vi "Send.vi"(8 "error in (no error)":errorcluster, 11 "BaseDriver in":refnum<class "BaseDriver.lvclass">) -> (0 "error out":errorcluster, 3 "BaseDriver out":refnum<class "BaseDriver.lvclass">)   [LabVIEW 2013, in "BaseDriver.lvclass"]
doc: "Send a message to the remote destination"
uses:
  BaseDriver.lvclass
  BaseDriver.lvclass/BaseDriver.ctl
  Reader/BaseReader/BaseReader.lvclass
  driver_state.ctl
  Message/BaseMessage/BaseMessage.lvclass/BaseMessage.ctl
  Responder/BaseResponder/BaseResponder.lvclass
  Message/BaseMessage/Read Timeout.vi
  Message/BaseMessage/BaseMessage.lvclass
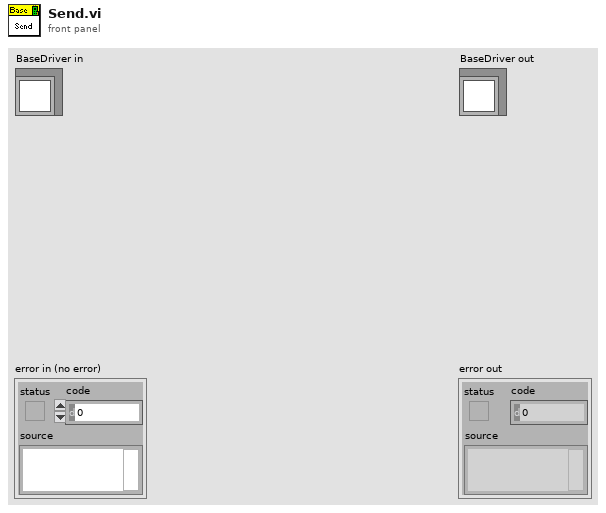
[diagram p1: front panel]
types:
  T1 = typedef "message_queue.ctl" = refnum<queue>
  T2 = typedef "driver_state.ctl" = enum16{"Idle", "Wait for ack"}
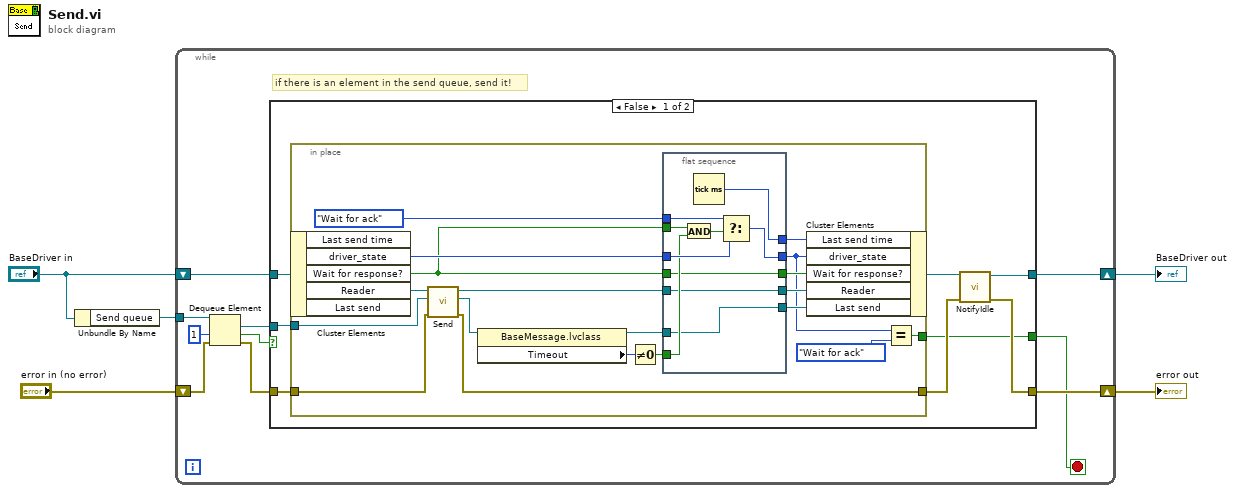
[diagram p0: block diagram]
diagram:
  n1 = Unbundle By Name("BaseDriver in") -> ("Send queue"=w3:T1)
  n2 = while {
    tunnel: w3 -> [w11]
    shift-right: [w8] -> w1
    shift-left: "BaseDriver in" -> [w12]
    shift-right: [w9] -> w2
    shift-left: "error in (no error)" -> [w13]
    stop <- w6 stop-if-true
    # "if there is an element in the send queue, send it!"
    n3 = Dequeue Element(queue=w11, timeout in ms (-1)=1, error in (no error)=w13) -> (element=w15:refnum<class "BaseMessage.lvclass">, timed out?=w7:bool, error out=w10:errorcluster)  [unwired: 1 out]
    n4 = case shown="False" w7 {
      selector: w7 -> [_ w54]
      tunnel: w15 -> [w23 _]
      tunnel: w12 -> [w22 w55]
      tunnel: [w19 w55] -> w8
      tunnel: w10 -> [w21 w53]
      tunnel: [w17 w53] -> w9
      tunnel: [w16 w54] -> w6
      frame False {
        n5 = in-place "In Place Element Structure" {
          in-place-border: w23 -> [w34]
          in-place-border: w21 -> [w39]
          in-place-border: [w24] -> w18
          in-place-border: [w26] -> w16
          n6 = in-place-cluster #1(w22) -> ("driver_state"=w40:T2, "Wait for response?"=w28:bool, "Reader"=w42:refnum<class "BaseReader.lvclass">)  [unwired: 2 out]
          n7 = call-dynamic "Send.vi"("error in (no error)"=w39, "Message"=w34, "BaseReader in"=w42) -> ("error out"=w24:errorcluster, "Sent Message"=w35:refnum<class "BaseMessage.lvclass">, "BaseReader out"=w30:refnum<class "BaseReader.lvclass">)  [unwired: 6 in]
          n8 = property on="Property Node" class="BaseMessage.lvclass"(reference=w35) -> (reference out=w32:refnum<class "BaseMessage.lvclass">, "Timeout"=w38:i32)  [unwired: 1 in, 1 out]
          n9 = Not Equal To 0?(x=w38) -> (x != 0?=w36:bool)
          n10 = flat-sequence {
            tunnel: driver_state."Wait for ack" ("driver_state") -> [w52]
            tunnel: w40 -> [w51]
            tunnel: [w50] -> w25
            tunnel: [w49] -> w37
            tunnel: w36 -> [w48]
            tunnel: w28 -> [w46]
            tunnel: [w45] -> w33
            tunnel: w32 -> [w45]
            tunnel: [w44] -> w31
            tunnel: w30 -> [w44]
            tunnel: [w43] -> w29
            tunnel: w28 -> [w43]
            frame #0 {
              n11 = And(x=w46, y=w48) -> (x .and. y?=w47:bool)
              n12 = Tick Count (ms)() -> (millisecond timer value=w49:u32)
              n13 = Select(t=w52, s=w47, f=w51) -> (s? t:f=w50:T2)
            }
          }
          n14 = in-place-cluster #1("Last send time"=w37, "driver_state"=w25, "Wait for response?"=w29, "Reader"=w31, "Last send"=w33) -> (w20:refnum<class "BaseDriver.lvclass">)
          n15 = Equal?(x=w25, y=driver_state."Wait for ack" ("x")) -> (x = y?=w26:bool)
        }
        n16 = call "NotifyIdle.vi"("error in (no error)"=w18, "BaseDriver in"=w20) -> ("error out"=w17:errorcluster, "BaseDriver out"=w19:refnum<class "BaseDriver.lvclass">)  [unwired: 8 in]
      }
      frame True {
      }
    }
  }
  "error out" <- w2
  "BaseDriver out" <- w1
